vi "GetBarcode 2DResultValue.vi"(8 "error in (no error)":errorcluster, 9 "data":T1, 11 "Analysis_Barcode 2D_Parameter":T2={"ROI"={"Global Rectangle"=[], "Contours"=[]}, "Barcode Type"=enum."PDF417", "Data Matrix Parameter"={"Data Matrix Description Options"={"Aspect Ratio"=0.0, "Rows"=0, "Columns"=0, "Rectangle"=FALSE, "ECC"=-2, "Barcode Polarity"=0, "Cell Fill Percentage"=-2, "Minimum Border Integrity %"=80.0, "Mirror Mode"=-2}, "Data Matrix Search Options"={"Rotation Mode"=enum."Unlimited", "Skip Location?"=FALSE, "Edge Threshold"=30, "Demodulation Mode"=-2, "Cell Sample Size"=-2, "Cell Filter Mode"=-2, "Skew Degrees Allowed"=5, "Maximum Iterations"=500, "Initial Search Vector Width"=5}, "Data Matrix Size Options"={"Data Matrix Size"={"Minimum Size"=0, "Maximum Size"=0}, "Quiet Zone Width"=10}, "Advanced Options"=[]}, "PDF147 Search Mode"=enum."Multiple Barcodes", "QR Code Parameter"={"QR Search Options"={"Rotation Mode"=enum."Unlimited", "Skip Location?"=FALSE, "Edge Threshold"=30, "Demodulation Mode"=-2, "Cell Sample Size"=-2, "Cell Filter Mode"=-2, "Skew Degrees Allowed"=5}, "QR Description Options"={"Matrix Size (cells)"=0, "Barcode Polarity"=-2, "Mirror Mode"=-2, "QR Model"=0}, "QR Code Cell Size (pixels)"={"Minimum Size"=3, "Maximum Size"=7}}} {"QR Code Parameter"."QR Description Options"."Mirror Mode" items=["Auto-detect"=-2, "Normal"=0, "Mirrored"=1]; "QR Code Parameter"."QR Description Options"."Matrix Size (cells)" items=["Auto-detect"=0, "11x11 - Version 1 (Micro QR Only)"=11, "13x13 - Version 2 (Micro QR Only)"=13, "15x15 - Version 3 (Micro QR Only)"=15, "17x17 - Version 4 (Micro QR Only)"=17, "21x21 - Version 1"=21, "25x25 - Version 2"=25, "29x29 - Version 3"=29, "33x33 - Version 4"=33, "37x37 - Version 5"=37, "41x41 - Version 6"=41, "45x45 - Version 7"=45, "49x49 - Version 8"=49, "53x53 - Version 9"=53, "57x57 - Version 10"=57, "61x61 - Version 11"=61, "65x65 - Version 12"=65, "69x69 - Version 13"=69, "73x73 - Version 14"=73, "77x77 - Version 15"=77, "81x81 - Version 16"=81, "85x85 - Version 17"=85, "89x89 - Version 18"=89, "93x93 - Version 19"=93, "97x97 - Version 20"=97, "101x101 - Version 21"=101, "105x105 - Version 22"=105, "109x109 - Version 23"=109, "113x113 - Version 24"=113, "117x117 - Version 25"=117, "121x121 - Version 26"=121, "125x125 - Version 27"=125, "129x129 - Version 28"=129, "133x133 - Version 29"=133, "137x137 - Version 30"=137, "141x141 - Version 31"=141, "145x145 - Version 32"=145, "149x149 - Version 33"=149, "153x153 - Version 34"=153, "157x157 - Version 35"=157, "161x161 - Version 36"=161, "165x165 - Version 37"=165, "169x169 -  Version 38"=169, "173x173 - Version 39"=173, "177x177 - Version 40"=177]; "QR Code Parameter"."QR Description Options"."QR Model" items=["Auto-detect", "Micro", "Model 1", "Model 2"]; "QR Code Parameter"."QR Description Options"."Barcode Polarity" items=["Auto-detect"=-2, "Black on White"=0, "White on Black"=1]; "QR Code Parameter"."QR Search Options"."Cell Filter Mode" items=["Auto-detect"=-2, "Average"=0, "Median"=1, "Central Average"=2, "High Average"=3, "Low Average"=4, "Very High Average"=5, "Very Low Average"=6, "All Filters"=8]; "QR Code Parameter"."QR Search Options"."Cell Sample Size" items=["Auto-detect"=-2, "1x1"=1, "2x2"=2, "3x3"=3, "4x4"=4, "5x5"=5, "6x6"=6, "7x7"=7]; "QR Code Parameter"."QR Search Options"."Demodulation Mode" items=["Auto-detect"=-2, "Histogram"=0, "Local Contrast"=1, "Combination"=2, "All"=3]; "Data Matrix Parameter"."Advanced Options"."Value" format="%.2f"; "Data Matrix Parameter"."Data Matrix Search Options"."Cell Filter Mode" items=["Auto-detect"=-2, "Average"=0, "Median"=1, "Central Average"=2, "High Average"=3, "Low Average"=4, "Very High Average"=5, "Very Low Average"=6, "All Filters"=8]; "Data Matrix Parameter"."Data Matrix Search Options"."Cell Sample Size" items=["Auto-detect"=-2, "1x1"=1, "2x2"=2, "3x3"=3, "4x4"=4, "5x5"=5, "6x6"=6, "7x7"=7]; "Data Matrix Parameter"."Data Matrix Search Options"."Demodulation Mode" items=["Auto-detect"=-2, "Histogram"=0, "Local Contrast"=1, "Combination"=2, "All"=3]; "Data Matrix Parameter"."Data Matrix Description Options"."Mirror Mode" items=["Auto-detect"=-2, "Normal"=0, "Mirrored"=1]; "Data Matrix Parameter"."Data Matrix Description Options"."ECC" items=["Auto-detect"=-2, "ECC 000"=0, "ECC 050"=50, "ECC 080"=80, "ECC 100"=100, "ECC 140"=140, "ECC 000-140"=190, "ECC 200"=200]; "Data Matrix Parameter"."Data Matrix Description Options"."Minimum Border Integrity %" format="%.2f"; "Data Matrix Parameter"."Data Matrix Description Options"."Aspect Ratio" format="%.2f"; "Data Matrix Parameter"."Data Matrix Description Options"."Cell Fill Percentage" items=["Auto-detect"=-2, "< 30%"=0, ">= 30%"=1]; "Data Matrix Parameter"."Data Matrix Description Options"."Barcode Polarity" items=["Auto-detect"=-2, "Black on White"=0, "White on Black"=1]}) -> (0 "error out":errorcluster, 3 "ResultValues":string[](array[string]))   [LabVIEW 2019]
uses:
  Controls/Barcode 2D/Analysis_Barcode 2D_Parameter.ctl
  <vilib>/vision/Instrument.llb/Data Matrix Description Options.ctl
  <vilib>/vision/Instrument.llb/ECC Type.ctl
  <vilib>/vision/Instrument.llb/Data Matrix Polarity.ctl
  <vilib>/vision/Instrument.llb/Cell Fill Percentage.ctl
  <vilib>/vision/Instrument.llb/Data Matrix Mirror.ctl
  <vilib>/vision/Instrument.llb/Data Matrix Search Options.ctl
  <vilib>/vision/Instrument.llb/Demodulation Mode.ctl
  <vilib>/vision/Instrument.llb/Cell Sample Size.ctl
  <vilib>/vision/Instrument.llb/Cell Filter Mode.ctl
  <vilib>/vision/Instrument.llb/Data Matrix Size Options.ctl
  <vilib>/vision/Instrument.llb/Data Matrix Advanced Options.ctl
  <vilib>/vision/Instrument.llb/QR Code Search Options.ctl
  <vilib>/vision/Instrument.llb/QR Code Description Options.ctl
  <vilib>/vision/Instrument.llb/QR Code Model Type.ctl
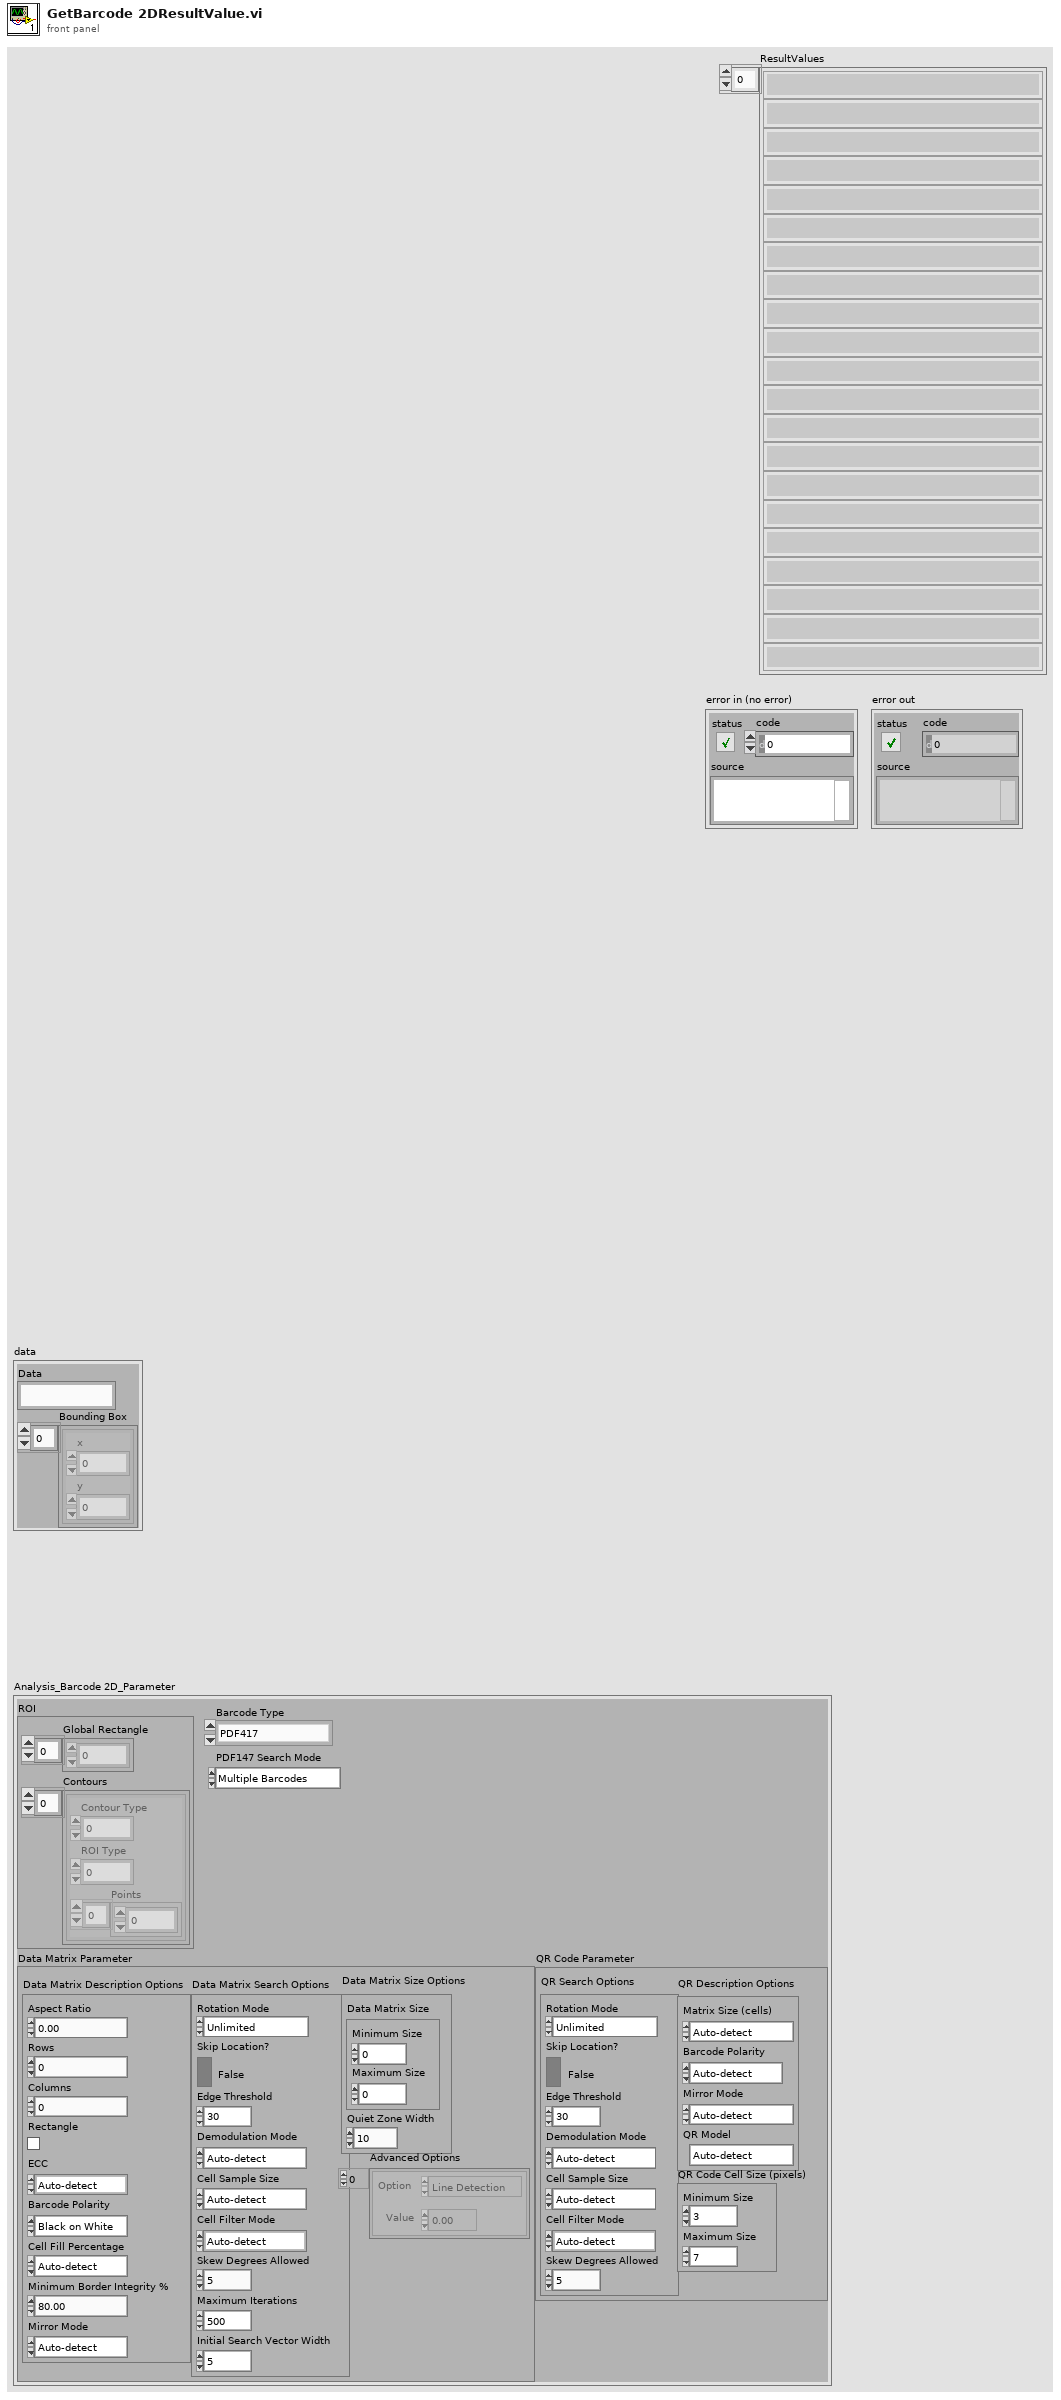
[diagram p1: front panel]
types:
  T1 = cluster{"Data":string, "Bounding Box":cluster{"x":sgl, "y":sgl}[]}
  T2 = typedef "Analysis_Barcode 2D_Parameter.ctl" = cluster{"ROI":cluster{"Global Rectangle":i32[], "Contours":cluster{"Contour Type":u32, "ROI Type":u32, "Points":i32[]}[]}, "Barcode Type":enum16{"Data Matrix", "PDF417", "QR Code"}, "Data Matrix Parameter":cluster{"Data Matrix Description Options":T3, "Data Matrix Search Options":T8, "Data Matrix Size Options":T12, "Advanced Options":T13[]}, "PDF147 Search Mode":T14, "QR Code Parameter":cluster{"QR Search Options":T15, "QR Description Options":T16, "QR Code Cell Size (pixels)":cluster{"Minimum Size":u32, "Maximum Size":u32}}}
  T3 = typedef "Data Matrix Description Options.ctl" = cluster{"Aspect Ratio":sgl, "Rows":u32, "Columns":u32, "Rectangle":bool, "ECC":T4, "Barcode Polarity":T5, "Cell Fill Percentage":T6, "Minimum Border Integrity %":sgl, "Mirror Mode":T7}
  T4 = typedef "ECC Type.ctl" = i32
  T5 = typedef "Data Matrix Polarity.ctl" = i32
  T6 = typedef "Cell Fill Percentage.ctl" = i32
  T7 = typedef "Data Matrix Mirror.ctl" = i32
  T8 = typedef "Data Matrix Search Options.ctl" = cluster{"Rotation Mode":enum32{"Unlimited", "0 Degrees", "90 Degrees", "180 Degrees", "270 Degrees"}, "Skip Location?":bool, "Edge Threshold":u32, "Demodulation Mode":T9, "Cell Sample Size":T10, "Cell Filter Mode":T11, "Skew Degrees Allowed":u32, "Maximum Iterations":u32, "Initial Search Vector Width":u32}
  T9 = typedef "Demodulation Mode.ctl" = i32
  T10 = typedef "Cell Sample Size.ctl" = i32
  T11 = typedef "Cell Filter Mode.ctl" = i32
  T12 = typedef "Data Matrix Size Options.ctl" = cluster{"Data Matrix Size":cluster{"Minimum Size":u32, "Maximum Size":u32}, "Quiet Zone Width":u32}
  T13 = typedef "Data Matrix Advanced Options.ctl" = cluster{"Option":enum32{"Line Detection", "HighLight Filter", "Aggressive", "FNC1", "Refine Bounding Box"}, " Value":dbl}
  T14 = typedef "PDF417 Search Mode" = enum32{"Multiple Barcodes", "Single Barcode, Conservative"}
  T15 = typedef "QR Code Search Options.ctl" = cluster{"Rotation Mode":enum32{"Unlimited", "0 Degrees", "90 Degrees", "180 Degrees", "270 Degrees"}, "Skip Location?":bool, "Edge Threshold":u32, "Demodulation Mode":T9, "Cell Sample Size":T10, "Cell Filter Mode":T11, "Skew Degrees Allowed":u32}
  T16 = typedef "QR Code Description Options.ctl" = cluster{"Matrix Size (cells)":i32, "Barcode Polarity":T5, "Mirror Mode":i32, "QR Model":T17}
  T17 = typedef "QR Code Model Type.ctl" = i32
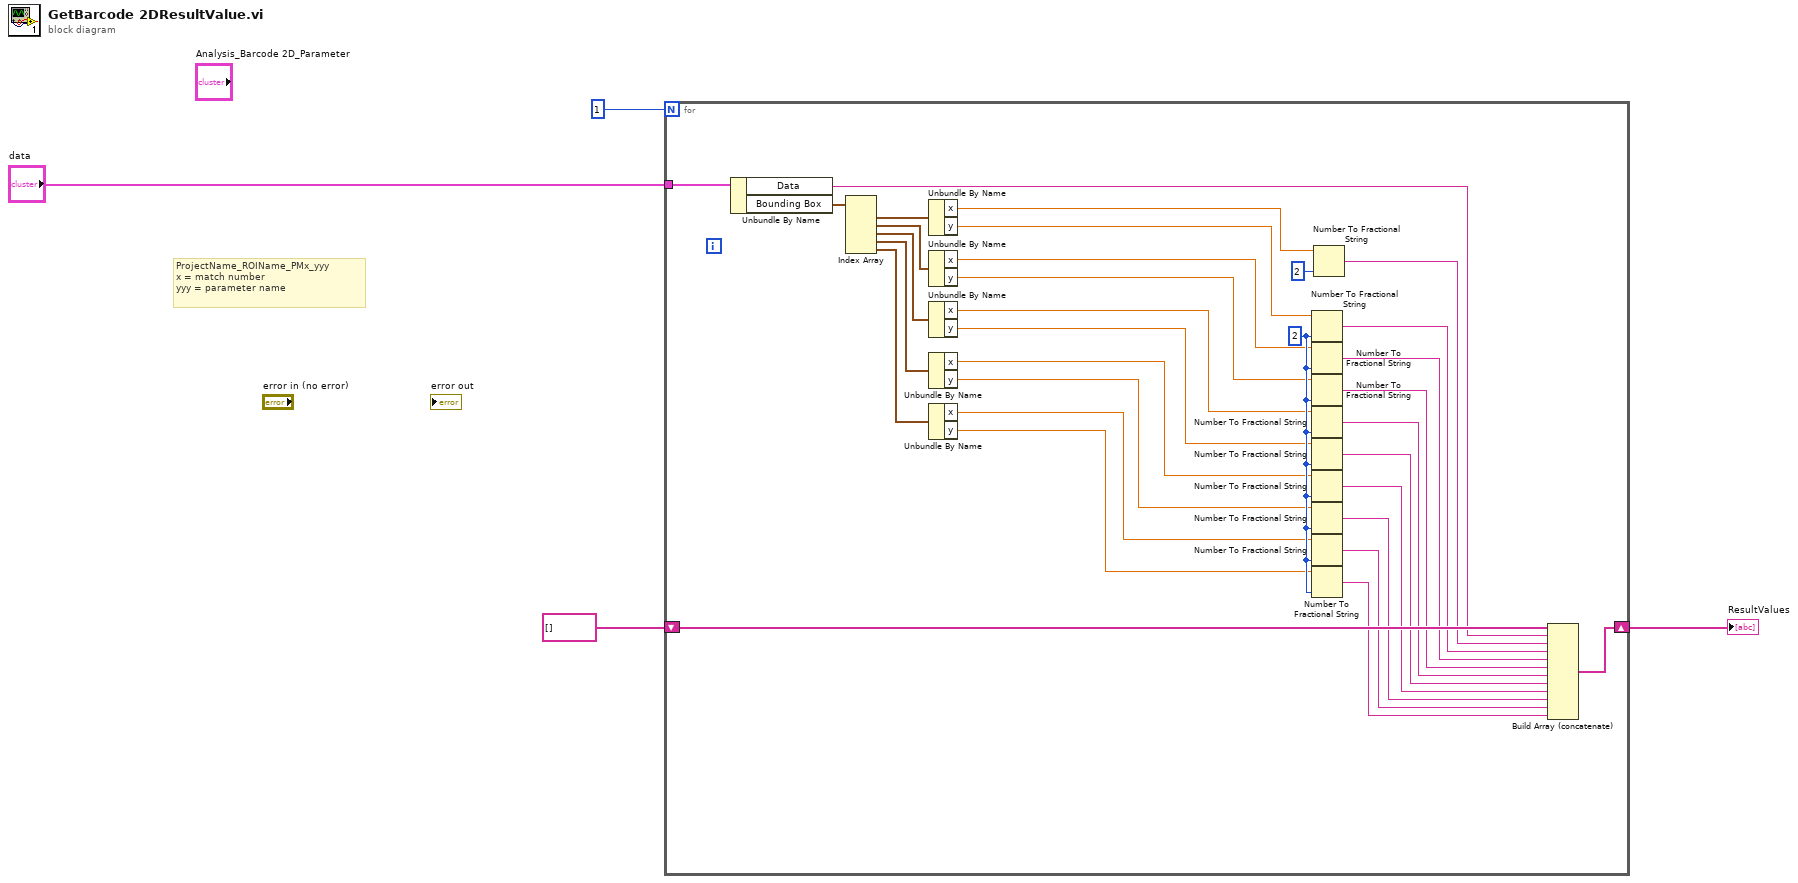
[diagram p0: block diagram]
diagram:
  # "ProjectName_ROIName_PMx_yyy\nx = match number\nyyy = parameter name"
  n1 = for {
    N: 1 -> [_]
    shift-right: [w34] -> w3
    shift-left: string[] [] -> [w35]
    tunnel: "data" -> [w36]
    w31 = i16 2 ("precision (6)")
    n2 = Unbundle By Name(w36) -> ("Data"=w15:string, "Bounding Box"=w21:cluster{"x":sgl, "y":sgl}[])
    n3 = Index Array(array=w21) -> (element #1=w20:cluster{"x":sgl, "y":sgl}, element #2=w19:cluster{"x":sgl, "y":sgl}, element #3=w18:cluster{"x":sgl, "y":sgl}, element #4=w17:cluster{"x":sgl, "y":sgl}, element #5=w16:cluster{"x":sgl, "y":sgl})  [unwired: 5 in]
    n4 = Unbundle By Name(w20) -> ("x"=w14:sgl, "y"=w13:sgl)
    n5 = Unbundle By Name(w19) -> ("x"=w12:sgl, "y"=w11:sgl)
    n6 = Unbundle By Name(w18) -> ("x"=w10:sgl, "y"=w9:sgl)
    n7 = Unbundle By Name(w17) -> ("x"=w8:sgl, "y"=w7:sgl)
    n8 = Unbundle By Name(w16) -> ("x"=w6:sgl, "y"=w5:sgl)
    n9 = Number To Fractional String(number=w13, precision (6)=w31) -> (F-format string=w30:string)  [unwired: 2 in]
    n10 = Number To Fractional String(number=w12, precision (6)=w31) -> (F-format string=w29:string)  [unwired: 2 in]
    n11 = Number To Fractional String(number=w11, precision (6)=w31) -> (F-format string=w28:string)  [unwired: 2 in]
    n12 = Number To Fractional String(number=w10, precision (6)=w31) -> (F-format string=w27:string)  [unwired: 2 in]
    n13 = Number To Fractional String(number=w9, precision (6)=w31) -> (F-format string=w26:string)  [unwired: 2 in]
    n14 = Number To Fractional String(number=w8, precision (6)=w31) -> (F-format string=w25:string)  [unwired: 2 in]
    n15 = Number To Fractional String(number=w7, precision (6)=w31) -> (F-format string=w24:string)  [unwired: 2 in]
    n16 = Number To Fractional String(number=w6, precision (6)=w31) -> (F-format string=w23:string)  [unwired: 2 in]
    n17 = Number To Fractional String(number=w5, precision (6)=w31) -> (F-format string=w22:string)  [unwired: 2 in]
    n18 = Number To Fractional String(number=w14, precision (6)=i16 2) -> (F-format string=w32:string)  [unwired: 2 in]
    n19 = Build Array (concatenate)(w35, w15, w32, w30, w29, w28, w27, w26, w25, w24, w23, w22) -> (w34:string[])
  }
  "ResultValues" <- w3
